vi "실습 5-1 클러스터.vi"(1 "클러스터":T2={"Input"=0.0, "Stop"=FALSE, "문자열"="", "배열"=[1.0, 2.0, 3.0, 4.0], "error in (no error)"={"status"=FALSE, "code"=0, "source"=""}}) -> (0 "클러스터 2":T1={"Output"=0.0, "Stop"=FALSE, "문자열"="", "배열"=[1.0, 2.0, 3.0, 4.0], "error in (no error)"={"status"=FALSE, "code"=0, "source"=""}})   [LabVIEW 2014]
panel:
  out "클러스터 4":T1={"Output"=0.0, "Stop"=FALSE, "문자열"="", "배열"=[1.0, 2.0, 3.0, 4.0], "error in (no error)"={"status"=FALSE, "code"=0, "source"=""}}
  in  "클러스터 3":T2={"Input"=0.0, "Stop"=FALSE, "문자열"="", "배열"=[1.0, 2.0, 3.0, 4.0], "error in (no error)"={"status"=FALSE, "code"=0, "source"=""}}
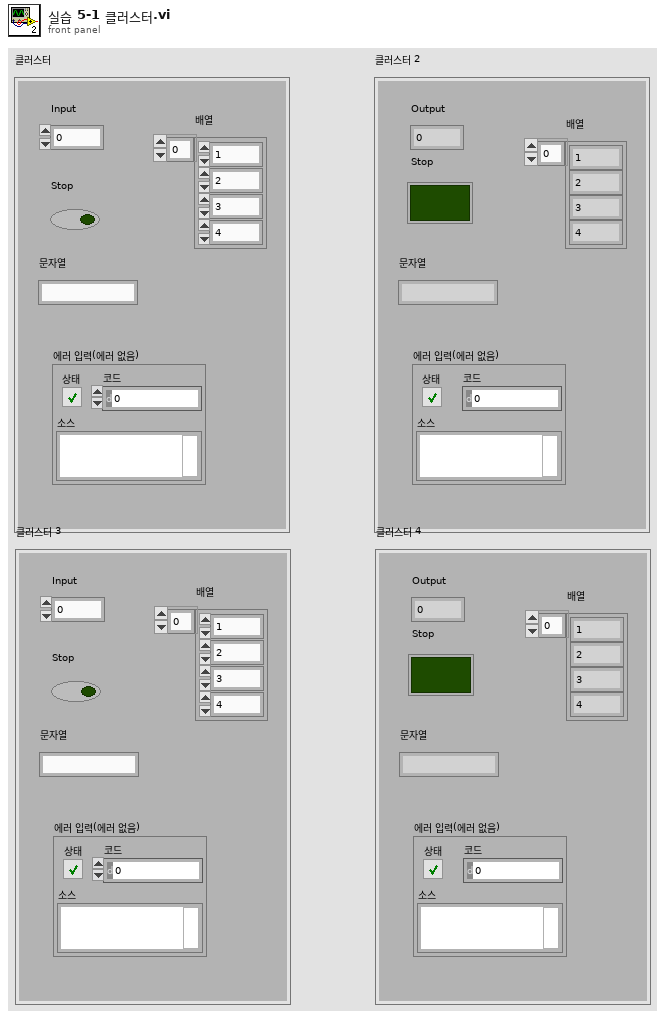
[diagram p1: front panel]
types:
  T1 = cluster{"Output":dbl, "Stop":bool, "문자열":string, "배열":dbl[], "error in (no error)":errorcluster}
  T2 = cluster{"Input":dbl, "Stop":bool, "문자열":string, "배열":dbl[], "error in (no error)":errorcluster}
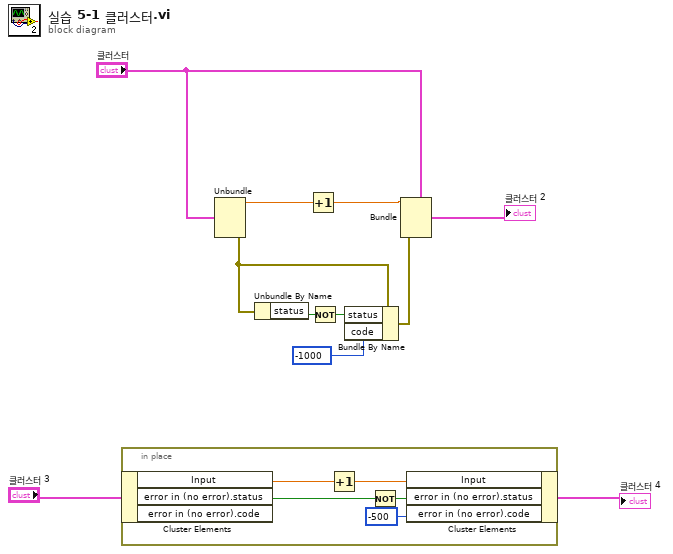
[diagram p0: block diagram]
diagram:
  n1 = in-place {
    n2 = in-place-cluster #1("클러스터 3") -> ("Input"=w16:dbl, "error in (no error).status"=w14:bool)  [unwired: 1 out]
    n3 = Increment(x=w16) -> (x+1=w15:dbl)
    n4 = Not(x=w14) -> (.not. x?=w13:bool)
    n5 = in-place-cluster #1("Input"=w15, "error in (no error).status"=w13, "error in (no error).code"=-500) -> (→"클러스터 4":T2)
  }
  n6 = Unbundle("클러스터") -> ("Input"=w9:dbl, "error in (no error)"=w7:errorcluster)  [unwired: 3 out]
  n7 = Unbundle By Name(w7) -> ("status"=w6:bool)
  n8 = Increment(x=w9) -> (x+1=w8:dbl)
  n9 = Not(x=w6) -> (.not. x?=w5:bool)
  n10 = Bundle By Name(cluster=w7, "status"=w5, "code"=-1000) -> (w4:errorcluster)
  n11 = Bundle(cluster="클러스터", "Input"=w8, "error in (no error)"=w4) -> (→"클러스터 2":T2)  [unwired: 3 in]
